vi "SetPageToTabCtrl.vi"(10 "index":i32, 11 "tab ctrl in":refnum<vi>) -> (3 "tab ctrl out":refnum<vi>)   [LabVIEW 2018, in "Library-Ctrl.lvlib"]
uses:
  Library-Ctrl.lvlib
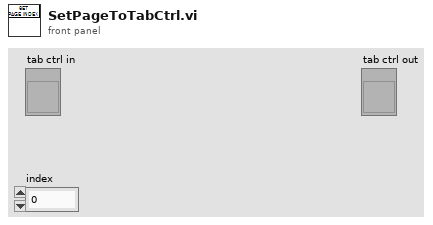
[diagram p1: front panel]
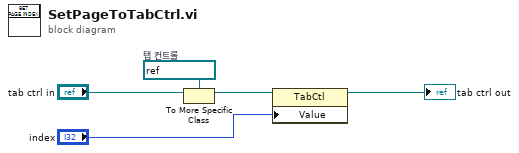
[diagram p0: block diagram]
diagram:
  w5 = refnum<vi> refnum  # 탭 컨트롤
  n1 = To More Specific Class(target class=w5, reference="tab ctrl in") -> (specific class reference=w4:refnum<vi>)  [unwired: 1 in, 1 out]
  n2 = property class="TabCtl"(reference=w4, "Value"="index") -> (reference out=→"tab ctrl out":refnum<vi>)  [unwired: 1 in, 1 out]
